vi "getSyncComponent.vi"(8 "error in (no error)":errorcluster, 11 "IDevice in":refnum<class "IDevice.lvclass">) -> (0 "error out":errorcluster, 2 "SyncComponent out":refnum<class "ISyncComponent.lvclass">, 3 "IDevice out":refnum<class "IDevice.lvclass">)   [LabVIEW 2022 SP3, in "openDAQ.lvlib" / "IBaseObject.lvlib" / "IPropertyObject.lvlib" / "IComponent.lvlib" / "IFolder.lvlib" / "IDevice.lvlib" / "IDevice.lvclass"]
uses:
  <instrlib>/openDAQ/Public/Classes/IDevice/IDevice.lvclass
  <instrlib>/openDAQ/Public/Classes/IDevice/IDevice.lvclass/IDevice.ctl
  <instrlib>/openDAQ/Public/Classes/ISyncComponent/ISyncComponent.lvclass
  <instrlib>/openDAQ/Binaries/Windows/x86/copendaq32.dll
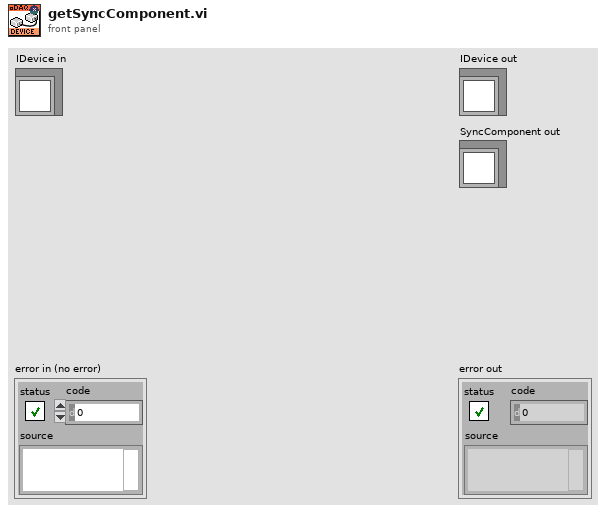
[diagram p1: front panel]
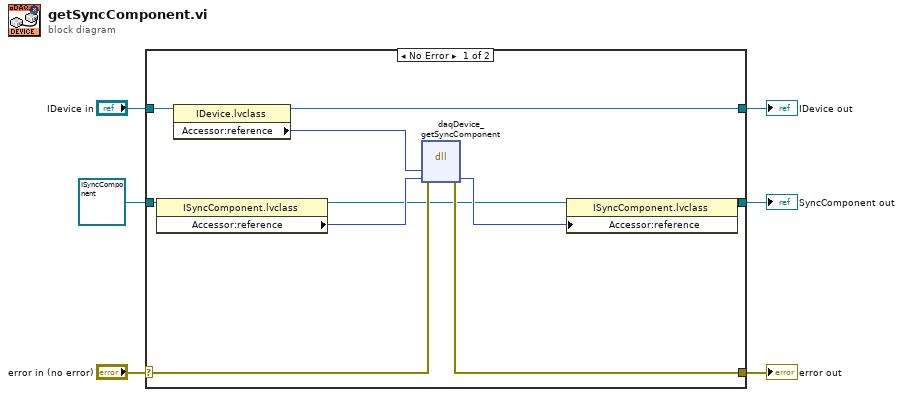
[diagram p0: block diagram]
diagram:
  n1 = case shown="No Error" "error in (no error)" {
    selector: "error in (no error)" -> [w15 w19]
    tunnel: [w14 w19] -> w5
    tunnel: [w9 w18] -> w3
    tunnel: "IDevice in" -> [w11 w18]
    tunnel: refnum<class "ISyncComponent.lvclass"> refnum ("openDAQ.lvlib:IBaseObject.lvlib:IPropertyObject.lvlib:IComponent.lvlib:ISyncComponent.lvlib:ISyncComponent.lvclass") -> [w8 w17]
    tunnel: [w7 w17] -> w1
    frame No Error {
      n2 = property class="ISyncComponent.lvclass"(reference=w8) -> (reference out=w12:refnum<class "ISyncComponent.lvclass">, "Accessor:reference"=w13:i64)  [unwired: 1 in, 1 out]
      n3 = property class="IDevice.lvclass"(reference=w11) -> (reference out=w9:refnum<class "IDevice.lvclass">, "Accessor:reference"=w10:i64)  [unwired: 1 in, 1 out]
      n4 = dll-call lib="C:/Program Files (x86)/National Instruments/LabVIEW 2022/instr.lib/openDAQ/Binaries/Windows/x86/copendaq*.*" fn="daqDevice_getSyncComponent"(error in=w15, "device"=w10, "syncComponent"=w13) -> (error out=w14:errorcluster, "syncComponent"=w16:i64)  [unwired: 4 in, 1 out]
      n5 = property class="ISyncComponent.lvclass"(reference=w12, "Accessor:reference"=w16) -> (reference out=w7:refnum<class "ISyncComponent.lvclass">)  [unwired: 1 in, 1 out]
    }
    frame Error {
    }
  }
  "error out" <- w5
  "IDevice out" <- w3
  "SyncComponent out" <- w1
